vi "Control Panel.vi"(8 "error in (no error)":errorcluster, 11 "Fake Wavelength Meter in":refnum<class "Wavelength Meter.lvclass">) -> (0 "error out":errorcluster, 3 "Fake Wavelength Meter out":refnum<class "Wavelength Meter.lvclass">)   [LabVIEW 2009, in "Wavelength Meter.lvclass"]
doc: "(Dynamic) A user-level application that simulates the physical front panel of the Instrument. Provide the user with buttons to manually control features of the instrument, and provide indicators of its current state."
uses:
  Wavelength Meter.lvclass
  HighFinesse WS5/Variable Typedefs.llb/Exposure Mode.ctl
  Utility Classes/Readable/Readable.lvclass
  Wavelength Meter.lvclass/Wavelength Meter.ctl
  HighFinesse WS5/HighFinesse WS5.lvlib
panel:
  out "Ready":bool
  out "Exposure (ms)":u16
  in  "Exposure Mode":T1
  in  "stop":bool
  in  "Read":bool
  in  "Set Exposure (ms)":u16
  out "Wavelength":dbl
  in  "Copy Actual to set":bool
  in  "Populate Fields with member data":bool
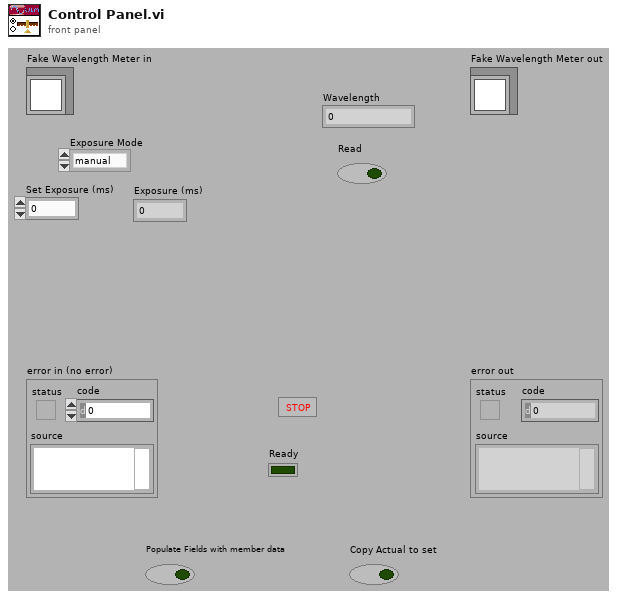
[diagram p1: front panel]
types:
  T1 = typedef "HighFinesse WS5.lvlib/Exposure Mode.ctl" = enum16{"manual", "automatic"}
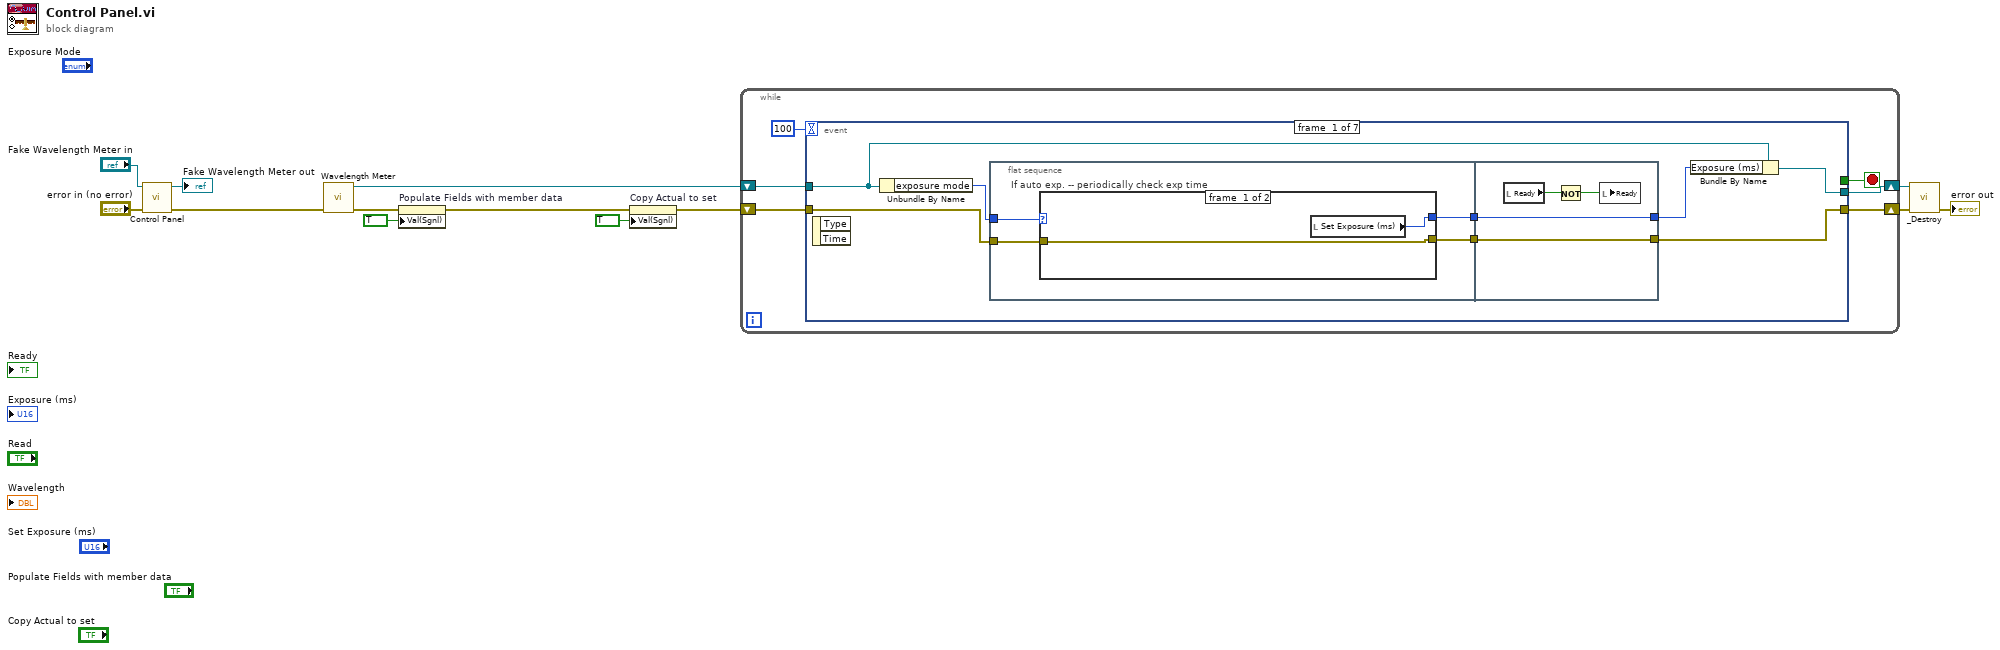
[diagram p0: block diagram]
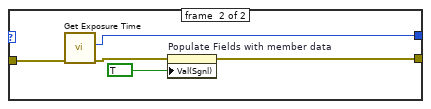
[diagram p2: hidden frame]
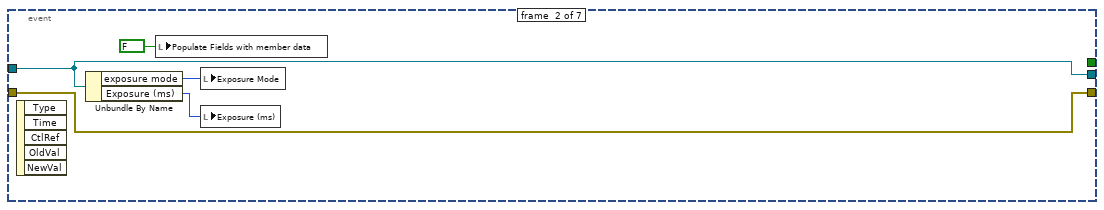
[diagram p3: hidden frame]
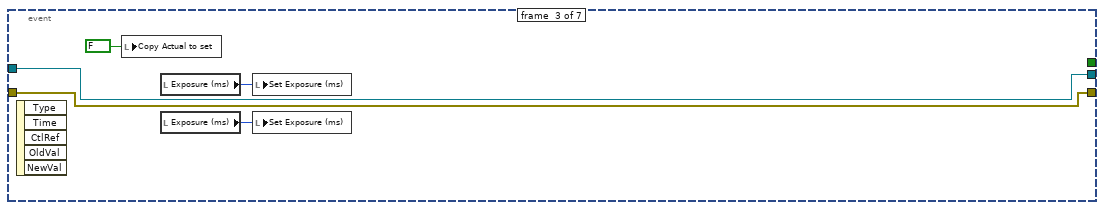
[diagram p4: hidden frame]
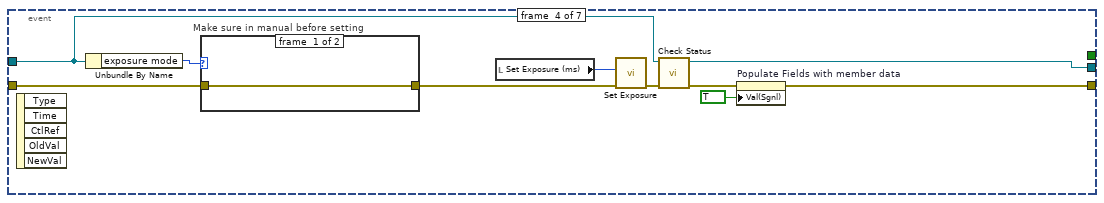
[diagram p5: hidden frame]
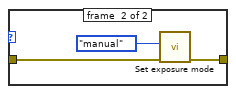
[diagram p6: hidden frame]
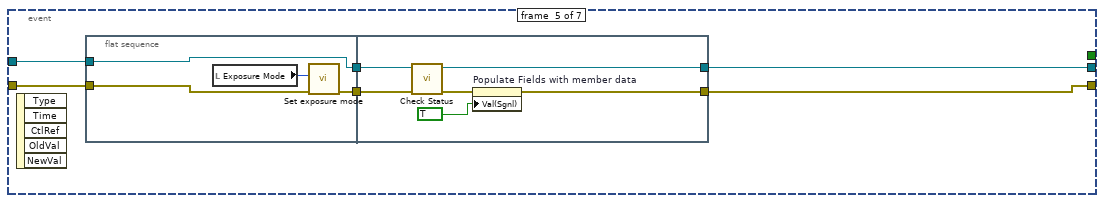
[diagram p7: hidden frame]
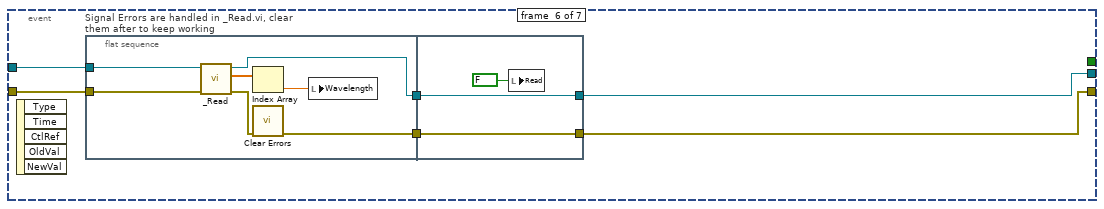
[diagram p8: hidden frame]
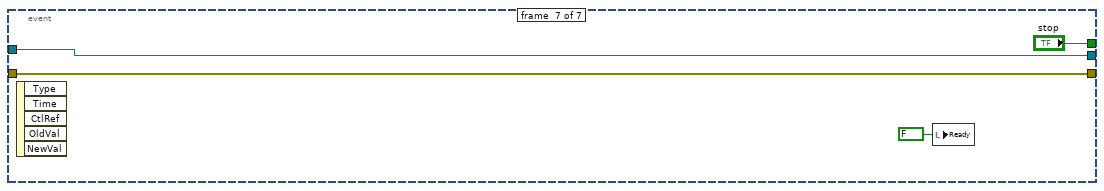
[diagram p9: hidden frame]
diagram:
  n1 = call-parent "Control Panel.vi"("error in (no error)"="error in (no error)", "Instrument in"="Fake Wavelength Meter in") -> ("error out"=w10:errorcluster, "Instrument out"=→"Fake Wavelength Meter out":refnum<class "Wavelength Meter.lvclass">)  [unwired: 8 in]
  n2 = call "Wavelength Meter.vi"("error in (no error)"=w10) -> ("error out"=w4:errorcluster, "Wavelength Meter out"=w8:refnum<class "Wavelength Meter.lvclass">)  [unwired: 9 in]
  n3 = property on="Populate Fields with member data" class="Bool (strict)"(error in=w4, "Val(Sgnl)"=TRUE ("Value (Signaling)")) -> (error out=w2:errorcluster)  [unwired: 1 in, 1 out]
  n4 = property on="Copy Actual to set" class="Bool (strict)"(error in=w2, "Val(Sgnl)"=TRUE ("Value (Signaling)")) -> (error out=w1:errorcluster)  [unwired: 1 in, 1 out]
  n5 = while {
    shift-right: [w18] -> w7
    shift-left: w8 -> [w19]
    shift-right: [w16] -> w6
    shift-left: w1 -> [w17]
    stop <- w15 stop-if-true
    n6 = event shown="[6] \"stop\": Value Change" {
      selector: _ -> [_ _ _ _ _ _ _]
      dyn-events: _ -> [_ _ _ _ _ _ _]
      timeout: 100 -> [_ _ _ _ _ _ _]
      tunnel: w19 -> [w24 w46 w52 w57 w69 w88 w101]
      tunnel: [w22 w46 w52 w56 w67 w86 w101] -> w18
      tunnel: [w25 w47 w51 w54 w70 w85 w100] -> w16
      tunnel: w17 -> [w26 w47 w51 w62 w72 w87 w100]
      tunnel: [_ _ _ _ _ _ "stop"] -> w15
      event #0 {
        n7 = event-data() -> ()  [unwired: 1 in, 2 out]
        n8 = Unbundle By Name(w24) -> ("exposure mode"=w27:T1)
        n9 = flat-sequence {
          tunnel: w27 -> [w31]
          tunnel: w26 -> [w30]
          tunnel: [w29] -> w21
          tunnel: [w28] -> w20
          tunnel: [w42] -> w23
          tunnel: [w39] -> w25
          tunnel: w21 -> [w39]
          tunnel: w20 -> [w42]
          frame #0 {
            n10 = case "If auto exp. -- periodically check exp time" shown="\"automatic\"" w31 {
              tunnel: w30 -> [w33 w38]
              tunnel: [w33 w34] -> w29
              tunnel: [w32 w37] -> w28
              frame #0 {
                n11 = local read "Set Exposure (ms)"() -> (w32:u16)
              }
              frame #1 {
                n12 = call "Get Exposure Time.vi"("error in (no error)"=w38) -> ("error out"=w35:errorcluster, "Exposure (ms)"=w37:u16)  [unwired: 9 in]
                n13 = property on="Populate Fields with member data" class="Bool (strict)"(error in=w35, "Val(Sgnl)"=TRUE ("Value (Signaling)")) -> (error out=w34:errorcluster)  [unwired: 1 in, 1 out]
              }
            }
          }
          frame #1 {
            n14 = local read "Ready"() -> (w41:bool)
            n15 = Not(x=w41) -> (.not. x?=w40:bool)
            n16 = local write "Ready"(w40) -> ()
          }
        }
        n17 = Bundle By Name(cluster=w24, "Exposure (ms)"=w23) -> (w22:refnum<class "Wavelength Meter.lvclass">)
      }
      event #1 {
        n18 = event-data() -> ()  [unwired: 1 in, 5 out]
        n19 = Unbundle By Name(w46) -> ("exposure mode"=w45:T1, "Exposure (ms)"=w44:u16)
        n20 = local write "Populate Fields with member data"(FALSE ("Populate Fields with member data")) -> ()
        n21 = local write "Exposure Mode"(w45) -> ()
        n22 = local write "Exposure (ms)"(w44) -> ()
      }
      event #2 {
        n23 = event-data() -> ()  [unwired: 1 in, 5 out]
        n24 = local write "Copy Actual to set"(FALSE ("Copy Actual to set")) -> ()
        n25 = local read "Exposure (ms)"() -> (w49:u16)
        n26 = local read "Exposure (ms)"() -> (w50:u16)
        n27 = local write "Set Exposure (ms)"(w49) -> ()
        n28 = local write "Set Exposure (ms)"(w50) -> ()
      }
      event #3 {
        n29 = event-data() -> ()  [unwired: 1 in, 5 out]
        n30 = Unbundle By Name(w57) -> ("exposure mode"=w61:T1)
        n31 = case "Make sure in manual before setting" shown="\"automatic\"" w61 {
          tunnel: w62 -> [w63 w66]
          tunnel: [w63 w65] -> w60
          frame #0 {
          }
          frame #1 {
            n32 = call "Set exposure mode.vi"("error in (no error)"=w66, "exposure mode"=Exposure_Mode."manual") -> ("error out"=w65:errorcluster)  [unwired: 8 in, 1 out]
          }
        }
        n33 = local read "Set Exposure (ms)"() -> (w59:u16)
        n34 = call "Set Exposure.vi"("error in (no error)"=w60, "Exposure (ms)"=w59) -> ("error out"=w58:errorcluster)  [unwired: 9 in]
        n35 = call-dynamic "Check Status.vi"("error in (no error)"=w58, "Wavelength Meter in"=w57) -> ("error out"=w55:errorcluster, "Wavelength Meter out"=w56:refnum<class "Wavelength Meter.lvclass">)  [unwired: 6 in, 2 out]
        n36 = property on="Populate Fields with member data" class="Bool (strict)"(error in=w55, "Val(Sgnl)"=TRUE ("Value (Signaling)")) -> (error out=w54:errorcluster)  [unwired: 1 in, 1 out]
      }
      event #4 {
        n37 = event-data() -> ()  [unwired: 1 in, 5 out]
        n38 = flat-sequence {
          tunnel: w72 -> [w76]
          tunnel: [w74] -> w71
          tunnel: w69 -> [w73]
          tunnel: [w73] -> w68
          tunnel: w71 -> [w82]
          tunnel: [w80] -> w70
          tunnel: w68 -> [w79]
          tunnel: [w78] -> w67
          frame #0 {
            n39 = local read "Exposure Mode"() -> (w75:T1)
            n40 = call "Set exposure mode.vi"("error in (no error)"=w76, "exposure mode"=w75) -> ("error out"=w74:errorcluster)  [unwired: 8 in, 1 out]
          }
          frame #1 {
            n41 = call-dynamic "Check Status.vi"("error in (no error)"=w82, "Wavelength Meter in"=w79) -> ("error out"=w81:errorcluster, "Wavelength Meter out"=w78:refnum<class "Wavelength Meter.lvclass">)  [unwired: 6 in, 2 out]
            n42 = property on="Populate Fields with member data" class="Bool (strict)"(error in=w81, "Val(Sgnl)"=TRUE ("Value (Signaling)")) -> (error out=w80:errorcluster)  [unwired: 1 in, 1 out]
          }
        }
      }
      event #5 {
        n43 = event-data() -> ()  [unwired: 1 in, 5 out]
        n44 = flat-sequence "Signal Errors are handled in _Read.vi, clear them after to keep working" {
          tunnel: w88 -> [w95]
          tunnel: w87 -> [w94]
          tunnel: [w91] -> w84
          tunnel: [w89] -> w83
          tunnel: [w97] -> w85
          tunnel: [w98] -> w86
          tunnel: w84 -> [w98]
          tunnel: w83 -> [w97]
          frame #0 {
            n45 = call-dynamic "_Read.vi"("error in (no error)"=w94, "Wavelength Meter in"=w95) -> ("error out"=w90:errorcluster, "4 Data Points"=w93:dbl[], "Wavelength Meter out"=w91:refnum<class "Wavelength Meter.lvclass">)  [unwired: 7 in]
            n46 = Index Array(array=w93) -> (element=w92:dbl)  [unwired: 1 in]
            n47 = call <vilib>:"Clear Errors.vi"("error in (no error)"=w90) -> ("error out"=w89:errorcluster)  [unwired: 6 in]
            n48 = local write "Wavelength"(w92) -> ()
          }
          frame #1 {
            n49 = local write "Read"(FALSE ("Read")) -> ()
          }
        }
      }
      event #6 {
        n50 = event-data() -> ()  [unwired: 1 in, 5 out]
        n51 = local write "Ready"(FALSE ("Ready")) -> ()
      }
    }
  }
  n52 = call-dynamic "_Destroy.vi"("error in (no error)"=w6, "Wavelength Meter in"=w7) -> ("error out"=→"error out":errorcluster)  [unwired: 9 in]
